vi "solar_log Filter.vi"(7 "LogIgnore":string[](array[string]), 10 "error in (no error)":errorcluster, 11 "MSG":string) -> (3 "Log?":bool)   [LabVIEW 2018]
doc: "This checks if the message is filter given the <b>Log Ignore</b> array. Use wildcards ('*') to filter messages. If an error exists the message is always logged regardless of the filter.\nEx: 'MyTarget:MyCMD' = 'MyTarget:*', '*:MyCMD', '*:*'"
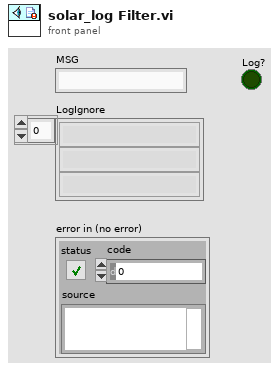
[diagram p1: front panel]
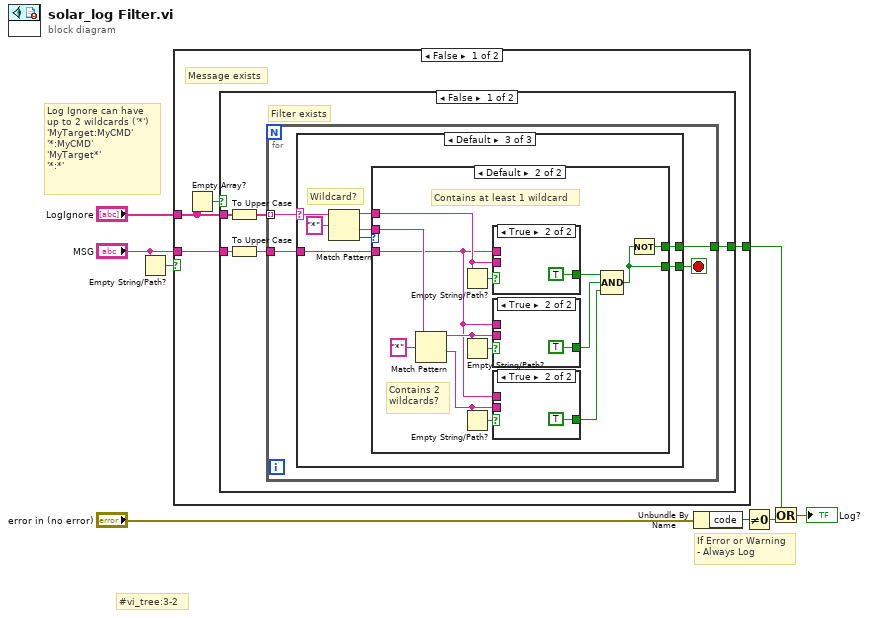
[diagram p0: block diagram]
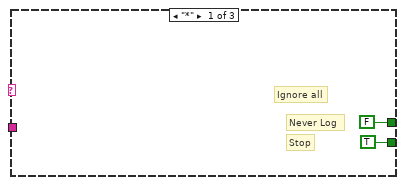
[diagram p2: hidden frame]
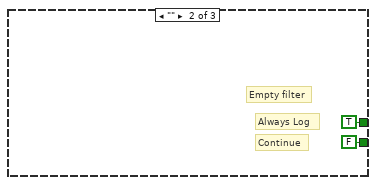
[diagram p3: hidden frame]
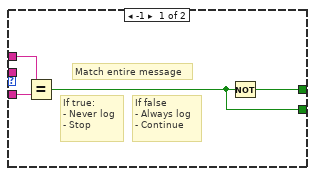
[diagram p4: hidden frame]
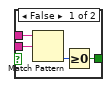
[diagram p5: hidden frame]
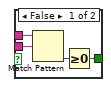
[diagram p6: hidden frame]
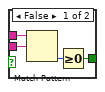
[diagram p7: hidden frame]
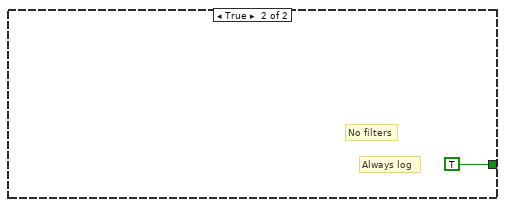
[diagram p8: hidden frame]
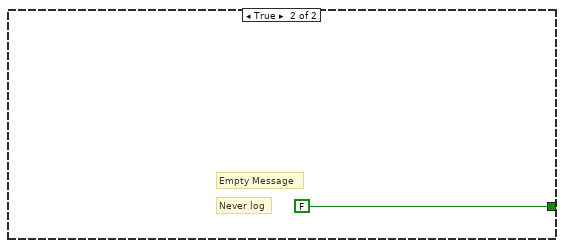
[diagram p9: hidden frame]
diagram:
  # "#vi_tree:3-2"
  # "Log Ignore can have\nup to 2 wildcards ('*')\n'MyTarget:MyCMD'\n'*:MyCMD'\n'MyTarget*'\n'*:*'"
  # "If Error or Warning\n- Always Log"
  n1 = Empty String/Path?(string/path="MSG") -> (empty?=w5:bool)
  n2 = case shown="False" w5 {
    tunnel: "LogIgnore" -> [w11 _]
    tunnel: "MSG" -> [w12 _]
    tunnel: [w9 FALSE] -> w2
    frame False {
      # "Message exists"
      n3 = Empty Array?(array=w11) -> (empty?=w10:bool)
      n4 = case shown="False" w10 {
        tunnel: w11 -> [w17 _]
        tunnel: w12 -> [w16 _]
        tunnel: [w13 TRUE] -> w9
        frame False {
          # "Filter exists"
          n5 = To Upper Case(1:w17) -> (0:w14:string[])
          n6 = To Upper Case(1:w16) -> (0:w15:string)
          n7 = for {
            tunnel: w14 -> [w20] mode=indexing
            tunnel: w15 -> [w21]
            tunnel: [w18] -> w13
            stop <- w19 stop-if-true
            n8 = case shown="Default" w20 {
              selector: w20 -> [_ _ w28]
              tunnel: w21 -> [_ _ w29]
              tunnel: [TRUE FALSE w27] -> w19
              tunnel: [FALSE TRUE w26] -> w18
              frame "*" {
                # "Stop"
                # "Never Log"
                # "Ignore all"
              }
              frame "" {
                # "Always Log"
                # "Continue"
                # "Empty filter"
              }
              frame Default {
                # "Wildcard?"
                n9 = Match Pattern(string=w28, regular expression="*") -> (before substring=w31:string, after substring=w30:string, offset past match=w32:i32)  [unwired: 1 in, 1 out]
                n10 = case shown="Default" w32 {
                  tunnel: w31 -> [w36 w51]
                  tunnel: w30 -> [_ w46]
                  tunnel: w29 -> [w37 w42]
                  tunnel: [w35 w40] -> w27
                  tunnel: [w34 w48] -> w26
                  frame -1 {
                    # "If false\n- Always log\n- Continue"
                    # "If true:\n- Never log\n- Stop"
                    # "Match entire message"
                    n11 = Equal?(x=w36, y=w37) -> (x = y?=w35:bool)
                    n12 = Not(x=w35) -> (.not. x?=w34:bool)
                  }
                  frame Default {
                    # "Contains 2 \nwildcards?"
                    # "Contains at least 1 wildcard"
                    n13 = Match Pattern(string=w46, regular expression="*") -> (before substring=w45:string, after substring=w43:string)  [unwired: 1 in, 2 out]
                    n14 = Empty String/Path?(string/path=w51) -> (empty?=w50:bool)
                    n15 = Empty String/Path?(string/path=w45) -> (empty?=w49:bool)
                    n16 = Empty String/Path?(string/path=w43) -> (empty?=w44:bool)
                    n17 = case shown="True" w50 {
                      tunnel: w51 -> [w65 _]
                      tunnel: w42 -> [w64 _]
                      tunnel: [w62 TRUE] -> w41
                      frame False {
                        n18 = Match Pattern(string=w64, regular expression=w65) -> (offset past match=w63:i32)  [unwired: 1 in, 3 out]
                        n19 = Greater Or Equal To 0?(x=w63) -> (x >= 0?=w62:bool)
                      }
                      frame True {
                      }
                    }
                    n20 = case shown="True" w49 {
                      tunnel: w45 -> [w60 _]
                      tunnel: w42 -> [w59 _]
                      tunnel: [w57 TRUE] -> w39
                      frame False {
                        n21 = Match Pattern(string=w59, regular expression=w60) -> (offset past match=w58:i32)  [unwired: 1 in, 3 out]
                        n22 = Greater Or Equal To 0?(x=w58) -> (x >= 0?=w57:bool)
                      }
                      frame True {
                      }
                    }
                    n23 = case shown="True" w44 {
                      tunnel: w43 -> [w55 _]
                      tunnel: w42 -> [w54 _]
                      tunnel: [w52 TRUE] -> w38
                      frame False {
                        n24 = Match Pattern(string=w54, regular expression=w55) -> (offset past match=w53:i32)  [unwired: 1 in, 3 out]
                        n25 = Greater Or Equal To 0?(x=w53) -> (x >= 0?=w52:bool)
                      }
                      frame True {
                      }
                    }
                    n26 = Compound Arithmetic op=AND(w41, w39, w38) -> (w40:bool)
                    n27 = Not(x=w40) -> (.not. x?=w48:bool)
                  }
                }
              }
            }
          }
        }
        frame True {
          # "Always log"
          # "No filters"
        }
      }
    }
    frame True {
      # "Empty Message"
      # "Never log"
    }
  }
  n28 = Unbundle By Name("error in (no error)") -> ("code"=w8:i32)
  n29 = Not Equal To 0?(x=w8) -> (x != 0?=w3:bool)
  n30 = Or(x=w2, y=w3) -> (x .or. y?=→"Log?":bool)
